vi "Begin.vi"   [LabVIEW 2014]
doc: "Called before other user functions, this VI is expected to open initial I/O refnums, load in file data, and do all program initialization. Notice that the <B>error out</B> terminal is simply used for data flow. Wiring it to other structures or subVIs ensures that this VI runs first."
uses:
  <vilib>/Rock Robotics/WPI/DriverStation/WPI_DriverStationRobotMode2.ctl
  Robot Global Data.vi
types:
  T1 = typedef "WPI_DriverStationRobotMode2.ctl" = enum16{"Autonomous Disabled", "Autonomous Enabled", "Teleop Disabled", "Teleop Enabled", "Disconnected", "Finish", "Test Disabled", "Test Enabled", "Emergency Stopped"}
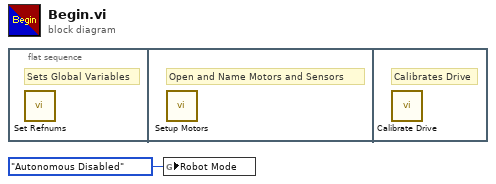
[diagram p0: block diagram]
diagram:
  n1 = flat-sequence {
    frame #0 {
      # "Sets Global Variables"
      n2 = call "Set Refnums.vi"() -> ()  [unwired: 12 in]
    }
    frame #1 {
      # "Open and Name Motors and Sensors"
      n3 = call "Setup Motors.vi"() -> ()  [unwired: 12 in]
    }
    frame #2 {
      # "Calibrates Drive"
      n4 = call "Calibrate Drive.vi"() -> ()  [unwired: 12 in]
    }
  }
  n5 = global write "Robot Global Data.vi" "Robot Mode"(WPI_DriverStationRobotMode2."Autonomous Disabled" ("Robot Mode")) -> ()
